vi "on_panel_resize.vi"(6 "PrevState":T2, 8 "error in (no error)":errorcluster, 9 "Act":T3=enum."Resized", 10 "NewBnds":T4, 11 "window in":refnum<class "rywindow.lvclass">) -> (0 "error out":errorcluster, 3 "window out":refnum<class "rywindow.lvclass">)   [LabVIEW 2017, in "rywindow.lvclass"]
uses:
  rywindow.lvclass
  <vilib>/Utility/miscctls.llb/LVRectTypeDef.ctl
  <vilib>/event_ctls.llb/sizeaction.ctl
  <vilib>/event_ctls.llb/panelstate.ctl
  <vilib>/Utility/miscctls.llb/LVBoundsTypeDef.ctl
  rywindow.lvclass/rywindow.ctl
  <vilib>/Utility/miscctls.llb/LVPositionTypeDef.ctl
panel:
  in  "Container Bounds":T1={"Width"=14, "Height"=23}
  out "iter":i32
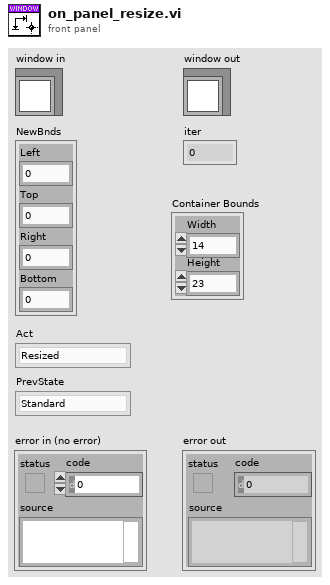
[diagram p1: front panel]
types:
  T1 = typedef "LVBoundsTypeDef.ctl" = cluster{"Width":u32, "Height":u32}
  T2 = typedef "panelstate.ctl" = enum32{"Standard", "Minimized", "Maximized"}
  T3 = typedef "sizeaction.ctl" = enum32{"Minimized", "Maximized", "Resized"}
  T4 = typedef "LVRectTypeDef.ctl" = cluster{"Left":i16, "Top":i16, "Right":i16, "Bottom":i16}
  T5 = typedef "LVPositionTypeDef.ctl" = cluster{"Left":i32, "Top":i32}
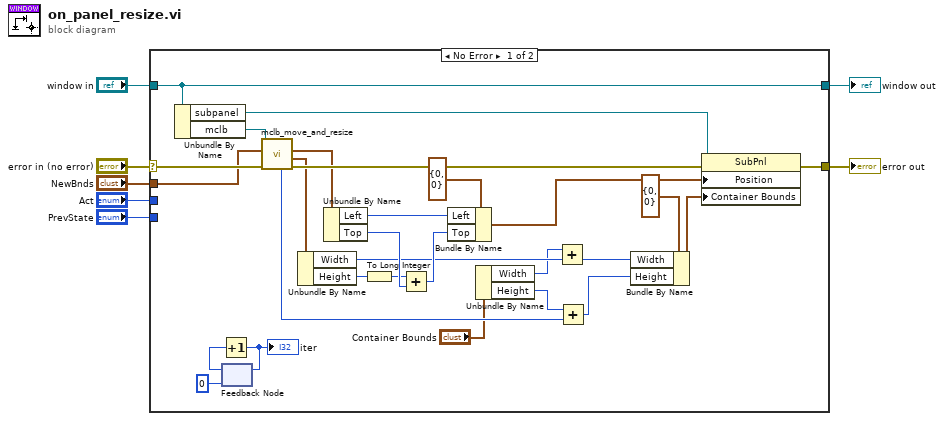
[diagram p0: block diagram]
diagram:
  n1 = case shown="No Error" "error in (no error)" {
    selector: "error in (no error)" -> [w34 w37]
    tunnel: [w27 w37] -> w6
    tunnel: [w35 w36] -> w4
    tunnel: "window in" -> [w35 w36]
    tunnel: "NewBnds" -> [w28 _]
    tunnel: "Act" -> [_ _]
    tunnel: "PrevState" -> [_ _]
    frame No Error {
      n2 = Unbundle By Name(w35) -> ("subpanel"=w26:refnum<vi>, "mclb"=w33:refnum<vi>)
      n3 = feedback #1(0) -> (w31:i32)
      n4 = Increment(x=w31) -> (x+1=w32:i32)
      "iter" <- w32
      n5 = feedback-in #1(w32) -> ()
      n6 = call "mclb_move_and_resize.vi"("error in (no error)"=w34, "Panel Resize.NewBnds"=w28, "mclb in"=w33) -> ("error out"=w29:errorcluster, "MCLB.Bounds"=w21:T1, "MCLB.Position"=w23:T5, "FP.Height"=w13:u32)  [unwired: 4 in, 1 out]
      n7 = Unbundle By Name(w21) -> ("Width"=w14:u32, "Height"=w20:u32)
      n8 = Unbundle By Name(w23) -> ("Left"=w22:i32, "Top"=w19:i32)
      n9 = To Long Integer(number=w20) -> (32bit integer=w17:i32)
      n10 = Add(x=w17, y=w19) -> (x+y=w18:i32)
      n11 = Bundle By Name(cluster=T5 {"Left"=0, "Top"=0} ("Position"), "Left"=w22, "Top"=w18) -> (w24:T5)
      n12 = Unbundle By Name("Container Bounds") -> ("Width"=w9:u32, "Height"=w8:u32)
      n13 = Add(x=w9, y=w14) -> (x+y=w11:u32)
      n14 = Add(x=w8, y=w13) -> (x+y=w12:u32)
      n15 = Bundle By Name(cluster=T1 {"Width"=0, "Height"=0} ("Container Bounds"), "Width"=w11, "Height"=w12) -> (w15:T1)
      n16 = property class="SubPnl"(reference=w26, error in=w29, "Position"=w24, "Container Bounds"=w15) -> (error out=w27:errorcluster)  [unwired: 1 out]
    }
    frame Error {
    }
  }
  "error out" <- w6
  "window out" <- w4
